vi "Set_Port_Status.vi"(6 "Byte 0":string(combo), 8 "error in (no error)":errorcluster, 9 "Byte 1":string(combo), 10 "CH":i32, 11 "Simulado in":refnum<class "Simulado.lvclass">) -> (0 "error out":errorcluster, 1 "Expected Response":string, 2 "Command to Send":string, 3 "Simulado out":refnum<class "Simulado.lvclass">)   [LabVIEW 2020, in "Simulado.lvclass"]
doc: "Arma el comando y una presupuestada respuesta para el comando de Set Port"
uses:
  Simulado.lvclass
  Abstract/Serial Device/Combo Box Comandos.ctl
  Abstract/Serial Device/Combo Box Devices.ctl
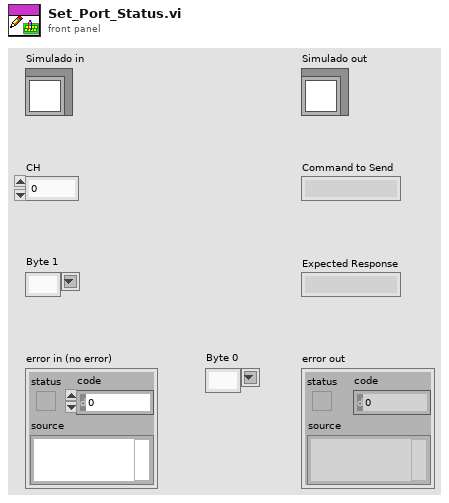
[diagram p1: front panel]
types:
  T1 = typedef "Combo Box Devices.ctl" = string
  T2 = typedef "Combo Box Comandos.ctl" = string
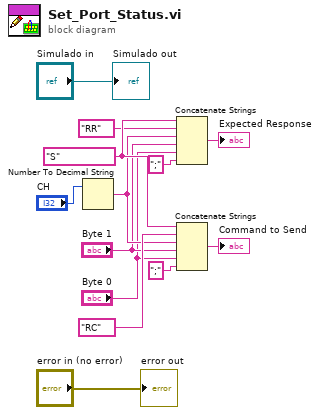
[diagram p0: block diagram]
diagram:
  w10 = T1 "S" ("Serial Devide Brand")
  n1 = Number To Decimal String(number="CH") -> (decimal integer string=w8:string)  [unwired: 1 in]
  n2 = Concatenate Strings(w10, T2 "RR" ("Respuesta"), w8, "Byte 1", "Byte 0", ";" ("string")) -> (→"Expected Response":string)
  n3 = Concatenate Strings(w10, T2 "RC" ("Command"), w8, "Byte 1", "Byte 0", ";" ("string")) -> (→"Command to Send":string)
  "error out" <- "error in (no error)"
  "Simulado out" <- "Simulado in"
